vi "Angle2Pos.vi"(10 "x":dbl) -> (2 "x/y":dbl)   [LabVIEW 2020]
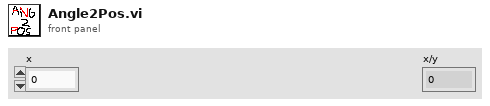
[diagram p1: front panel]
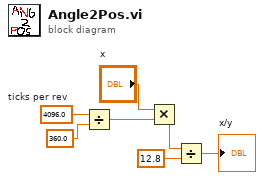
[diagram p0: block diagram]
diagram:
  w6 = 4096.0  # ticks per rev
  n1 = Divide(x=w6, y=360.0) -> (x/y=w7:dbl)
  n2 = Multiply(x="x", y=w7) -> (x*y=w3:dbl)
  n3 = Divide(x=w3, y=12.8) -> (x/y=→"x/y":dbl)
